vi "Generate X Ramp.vi"(1 "Map geometry out":T1) -> (0 "Ramp Pattern":dbl[](array[numeric]))   [LabVIEW 2010]
uses:
  <vilib>/Analysis/1siggen.llb/Ramp Pattern by Delta.vi
  <vilib>/Analysis/NI_AALBase.lvlib
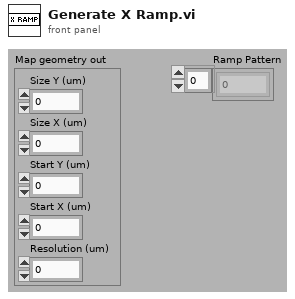
[diagram p1: front panel]
types:
  T1 = cluster{"Size Y (um)":dbl, "Size X (um)":dbl, "Start Y (um)":dbl, "Start X (um)":dbl, "Resolution (um)":dbl}
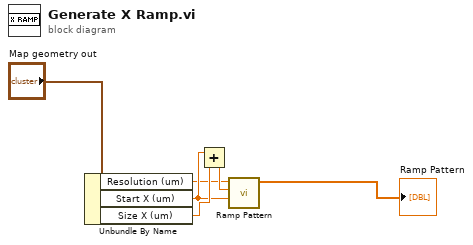
[diagram p0: block diagram]
diagram:
  n1 = Unbundle By Name("Map geometry out") -> ("Resolution (um)"=w1:dbl, "Start X (um)"=w3:dbl, "Size X (um)"=w4:dbl)
  n2 = Add(x=w3, y=w4) -> (x+y=w5:dbl)
  n3 = call-poly <vilib>:"Ramp Pattern.vi"("start"=w3, "end"=w5, "delta"=w1) -> ("Ramp Pattern"=→"Ramp Pattern":dbl[])  [unwired: 6 in, 2 out]
